vi "RunTest2.vi"(8 "error in (no error)":errorcluster, 11 "Prueba06 in":refnum<class "Prueba06.lvclass">) -> (0 "error out":errorcluster, 2 "resultado":string, 3 "Prueba06 out":refnum<class "Prueba06.lvclass">)   [LabVIEW 2019]
uses:
  Control/EstadosP06.ctl
  Prueba06.lvclass
  Control/MessageP06.ctl
  <vilib>/Utility/miscctls.llb/LVRowAndColumnTypeDef.ctl
  Prueba/Prueba.lvclass
  Prueba04/Control/Slide.ctl
  Prueba04/Prueba04.lvclass
  QMH/User Event - Stop/User Event - Stop.lvlib
  QMH/Message Queue/Message Queue.lvlib
  QMH/Message Queue/Enqueue Message (Single).vi
  ClusterGEN.ctl
  <vilib>/Utility/error.llb/Error Cluster From Error Code.vi
  <vilib>/ErrorRing/Error Ring.xnode
  <vilib>/Utility/error.llb/DialogType.ctl
  D:/REPO/GitHub/procal/Pruebas/Prueba/Prueba.lvclass
panel:
  out "tipoPrueba":string
  out "filaSelecc":i32
  out "TablaVoltajes":string[](array[string])
  out "cumple_no_cumple":bool
  out "n° filas":i32
  out "ptoCentral":dbl=2.0 format="%#.1f"
  out "Vref":dbl
  in  "Tab":enum32{"Page 1", "Page 2"}(tab)
  out "RangoRef":string
  out "frecuencia1":dbl=140.0
  in  "guardar_Vref":bool
  out "nivelRef":dbl=95.0 format="%.1f"
  in  "generar1":bool
  in  "AjusteAmp":T1=50.0 caption="Ajuste de amplitud [mV]" scale=0.0..20000.0
  out "voltaje1":dbl format="%.1f"
  out "frecuencia1":dbl format="%.1f"
  in  "seguir":bool
  out "Pict Ring 3":u16(ring)
  out "Pict Ring 2":u16(ring)
  in  "generar2":bool caption="PruebaSup"
  in  "PruebaInf":bool caption="PruebaSup"
  in  "PruebaSup":bool
  in  "Tabla":string[][](table)
  in  "salir":bool
  out "cumple":bool
  out "no_cumple":bool
  out "voltaje2":dbl format="%.1f"
  out "frecuencia2":dbl format="%.1f"
  in  "cb_rangoRef":string(combo)="1000"
  out "RangoRef2":string
  # "Elección Señal de Referencia\nsegún marca y modelo de sonómetro"
  # "Nivel Señal Referencia"
  # "Rango Referencia"
  # "Frecuencia"
  # "Monitoreo"
  # "Frecuencia"
  # "Hz"
  # "Voltaje"
  # "mV"
  # "6. Linealidad de nivel en el rango de referencia. IEC 61672-3: 2006 Cláusula 14"
  # "Tabla Resultados"
  # "Rango [dBA]"
  # "Referencia [dBA]"
  # "Cumple"
  # "No Cumple"
  # "6. Linealidad de nivel en el rango de referencia. IEC 61672-3: 2006 Cláusula 14"
  # "Monitoreo"
  # "Frecuencia"
  # "Hz"
  # "Voltaje"
  # "mV"
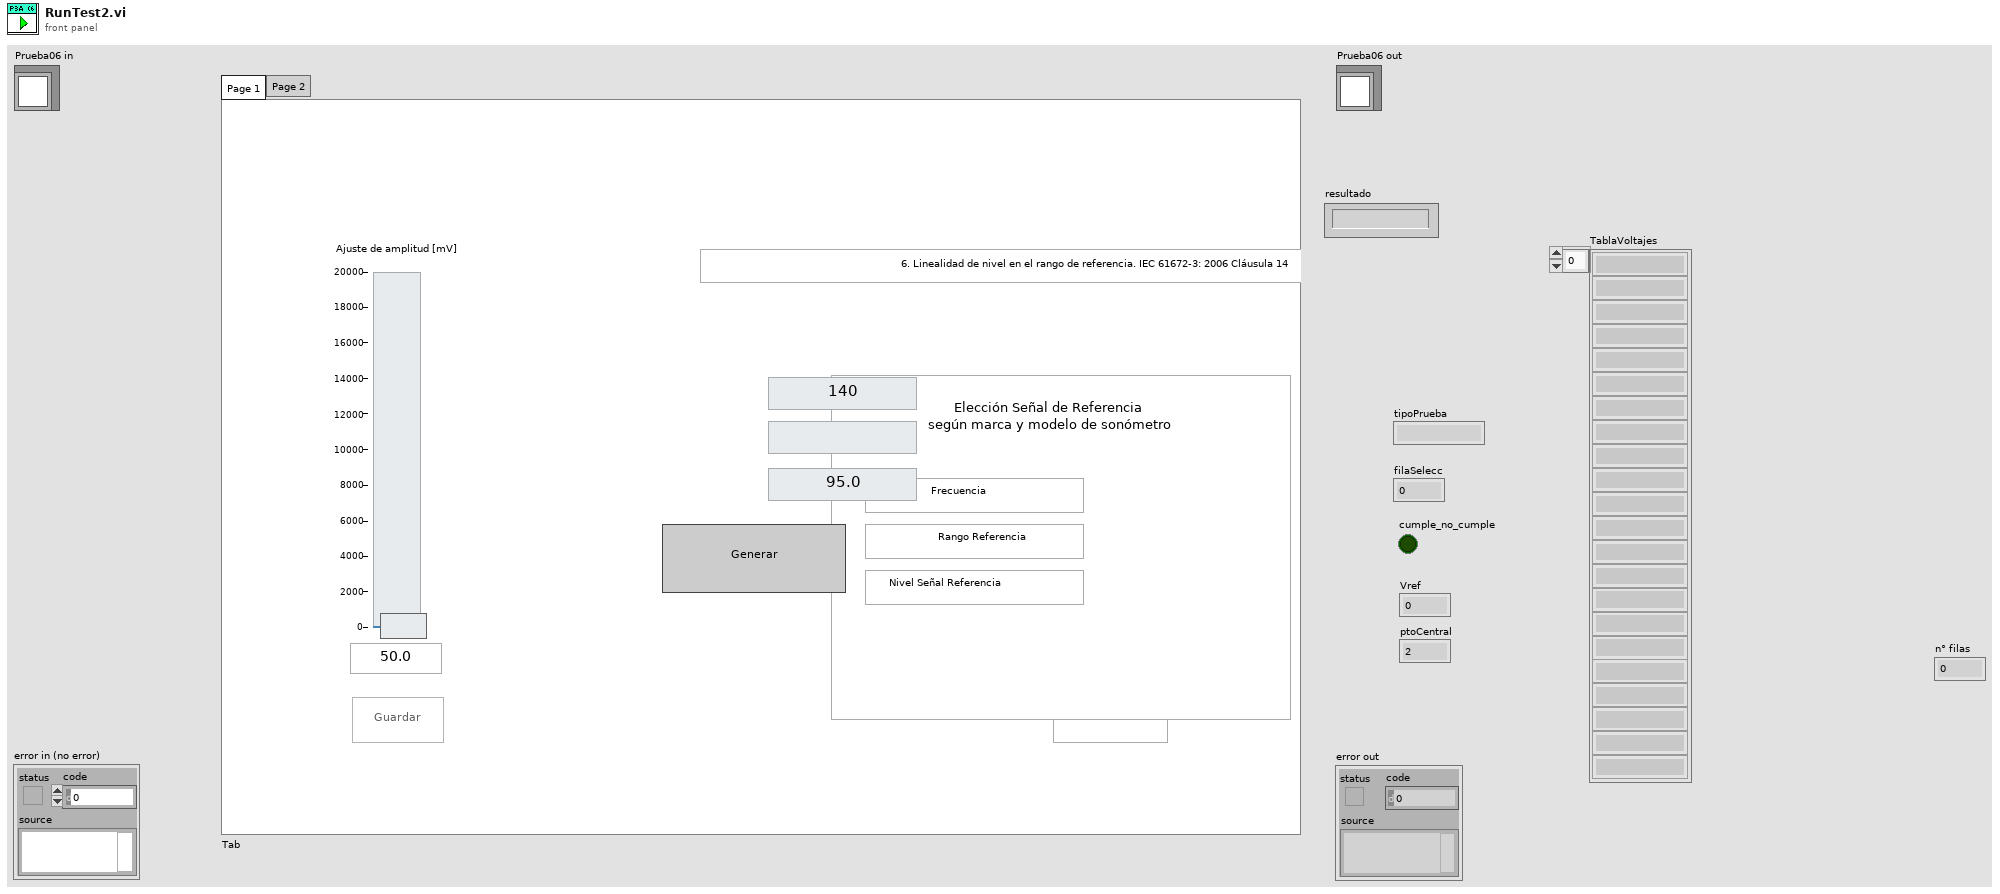
[diagram p1: front panel]
types:
  T1 = typedef "Prueba04.lvclass/Slide.ctl" = dbl
  T2 = typedef "LVRowAndColumnTypeDef.ctl" = cluster{"Row":i32, "Column":i32}
  T3 = typedef "Message Queue.lvlib/All Message Queues.ctl" = cluster{"MHL":refnum<queue>, "Inst_CNT90":refnum<queue>, "Inst_DS360":refnum<queue>, "Inst_Keithley2002":refnum<queue>, "Inst_DAQ":refnum<queue>, "BD":refnum<queue>, "Pistofono":refnum<queue>, "Nexus":refnum<queue>}
  T4 = enum8{"Enabled", "Disabled", "Disabled and Grayed Out"}
  T5 = typedef "Prueba06.lvclass/MessageP06.ctl" = cluster{"Estado":T6, "Data":variant}
  T6 = typedef "Prueba06.lvclass/EstadosP06.ctl" = enum16{"inicio", "LeerArchivoConfiguracion", "ConfirmarSalida", "DetieneInstrumentos", "InicializaInstrumento", "leerRango", "configuraRango", "calcularVref", "configuraTabla", "FrecAmp1", "FrecAmp2", "iniciarGEN", "monitoreo", "detenerGEN", "ajusteAmp", "guardaVerf", "creaVoltPrueba", "preguntaTipoPrueba", "guardarMediciones", "ingresaMediciones", "cumplimiento", "listo_evaluar", "evaluar", "final", "salir"}
  T7 = enum32{"Page 1", "Page 2", "Page 3", "Page 4", "Page 5", "Page 6", "Page 7"}
  T8 = typedef "Prueba06.lvclass/ClusterGEN.ctl" = cluster{"frec":dbl, "amp":dbl}
  T9 = cluster{"ControlName":string, "ControlReference":refnum<vi>}[]
  T10 = typedef "DialogType.ctl" = u16
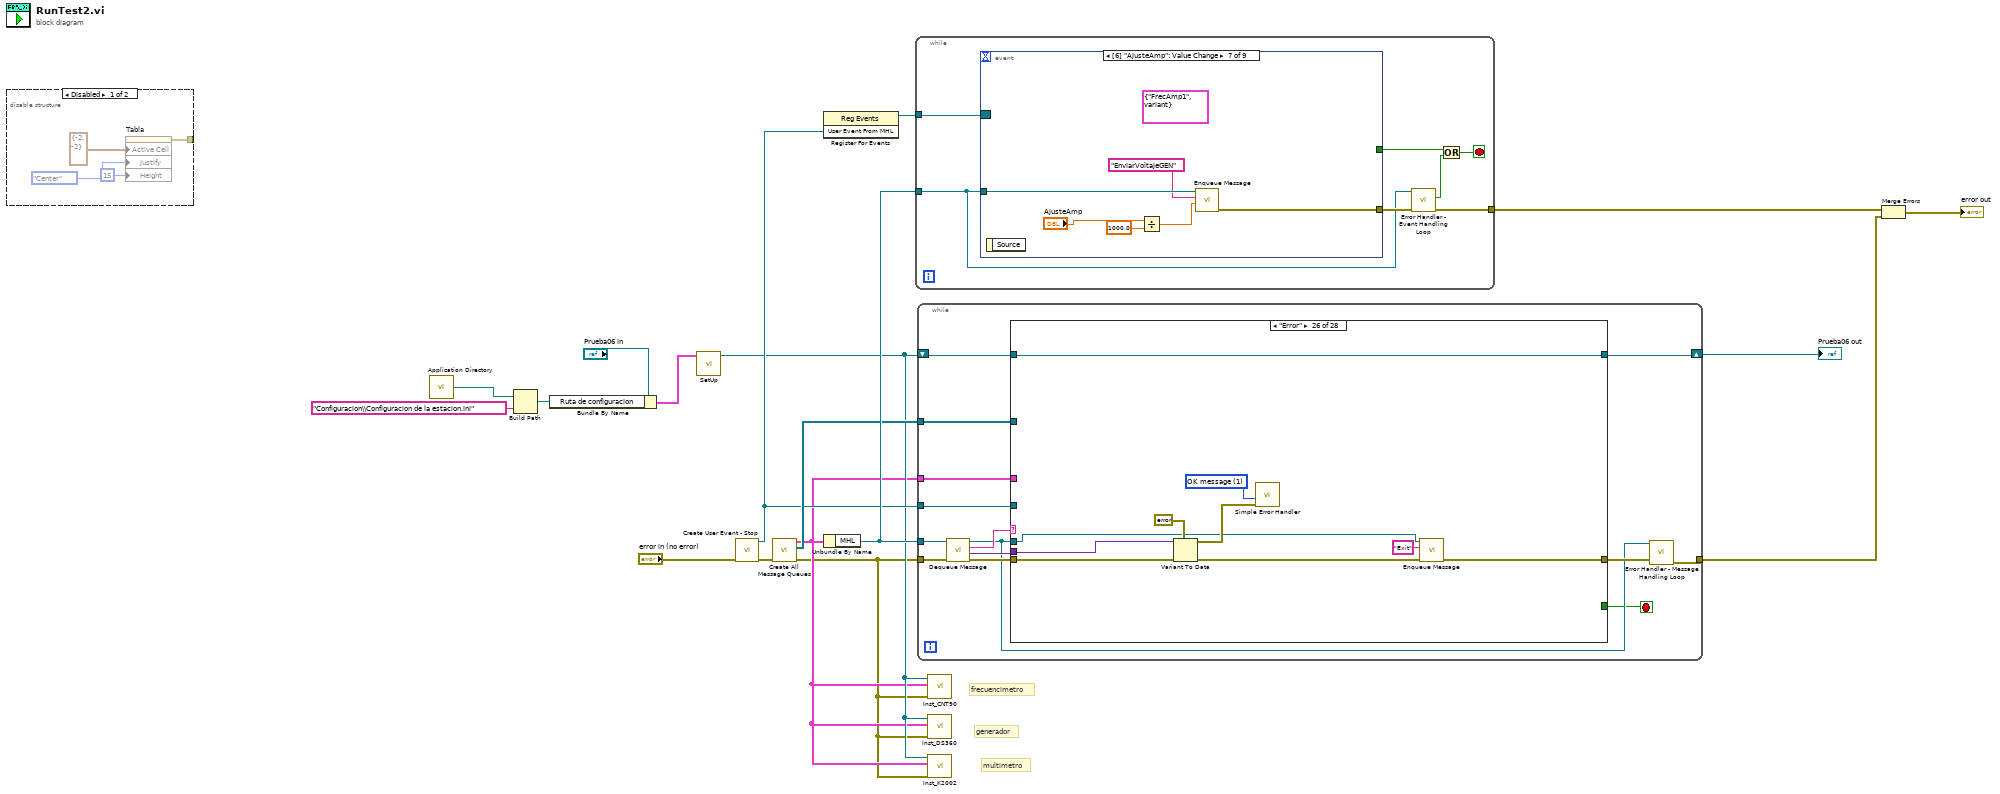
[diagram p0: block diagram]
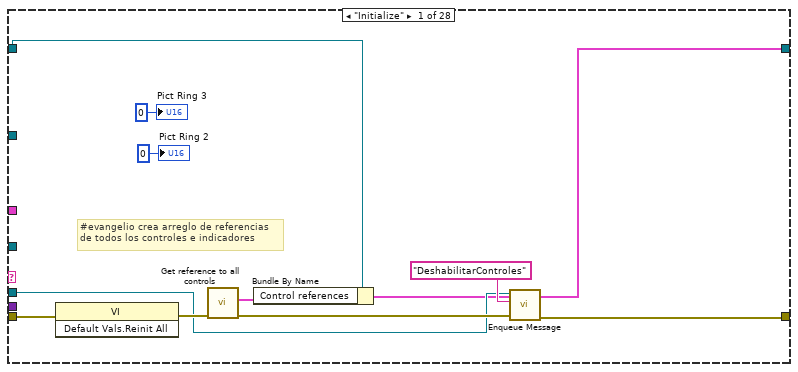
[diagram p3: hidden frame]
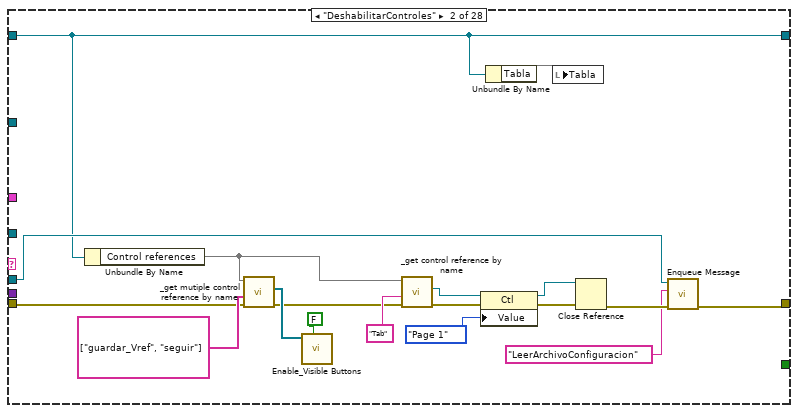
[diagram p4: hidden frame]
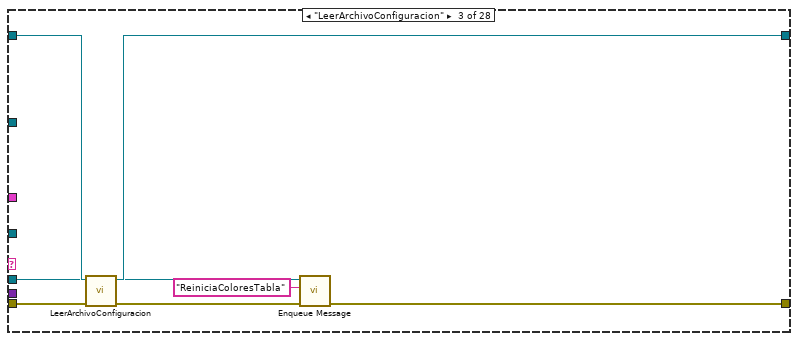
[diagram p5: hidden frame]
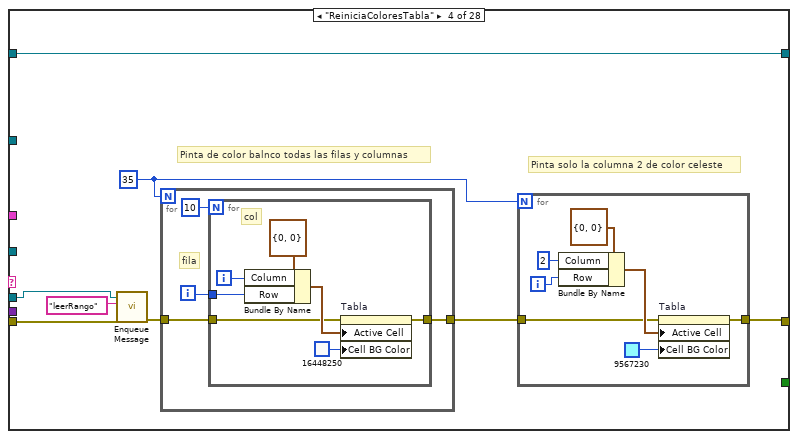
[diagram p6: hidden frame]
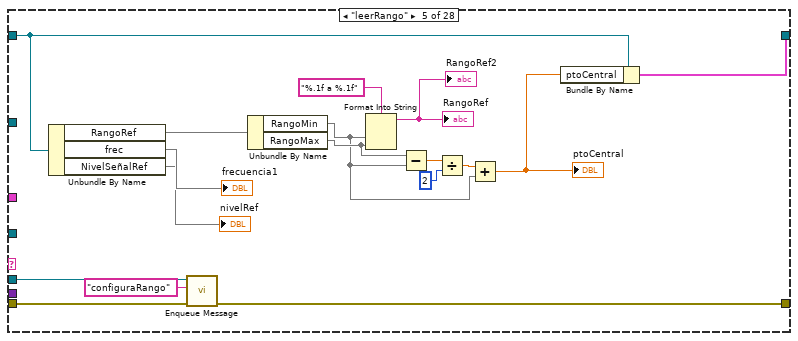
[diagram p7: hidden frame]
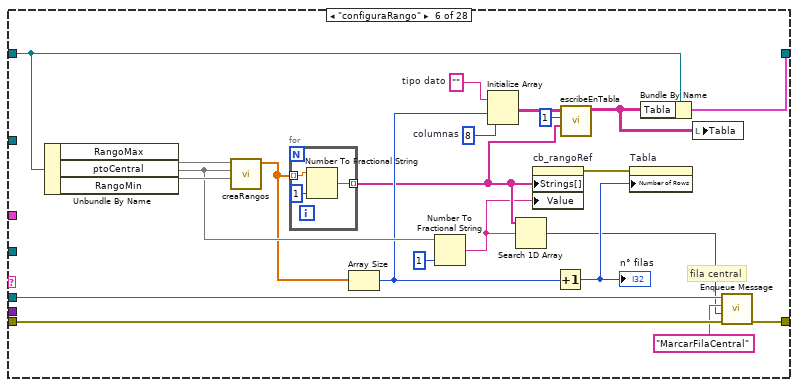
[diagram p8: hidden frame]
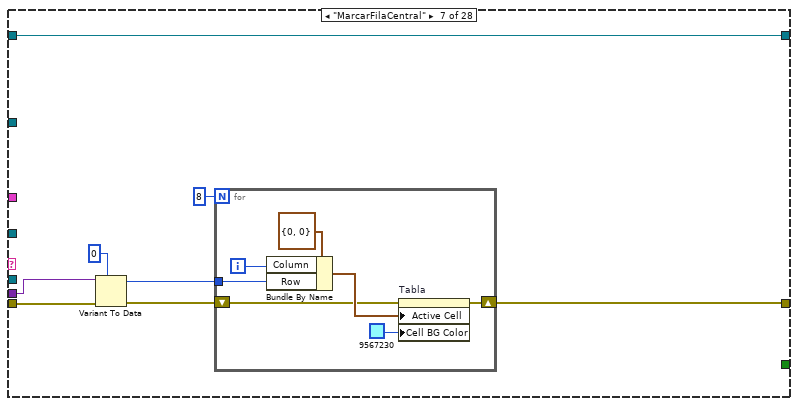
[diagram p9: hidden frame]
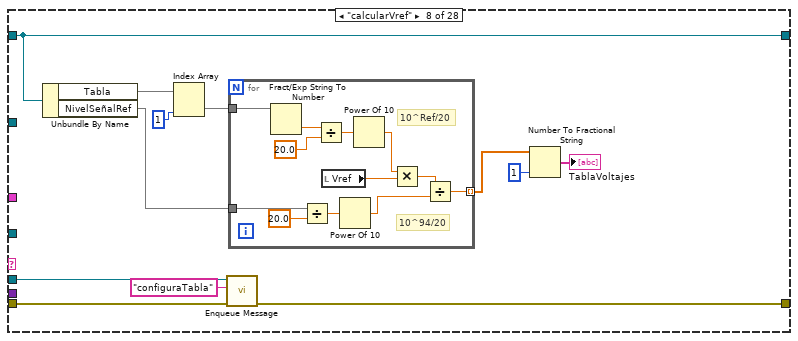
[diagram p10: hidden frame]
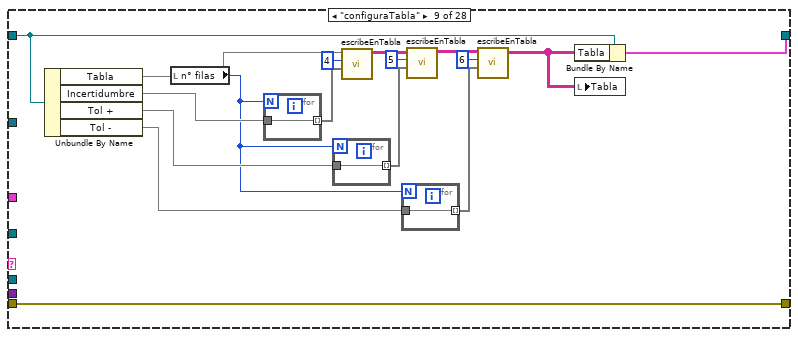
[diagram p11: hidden frame]
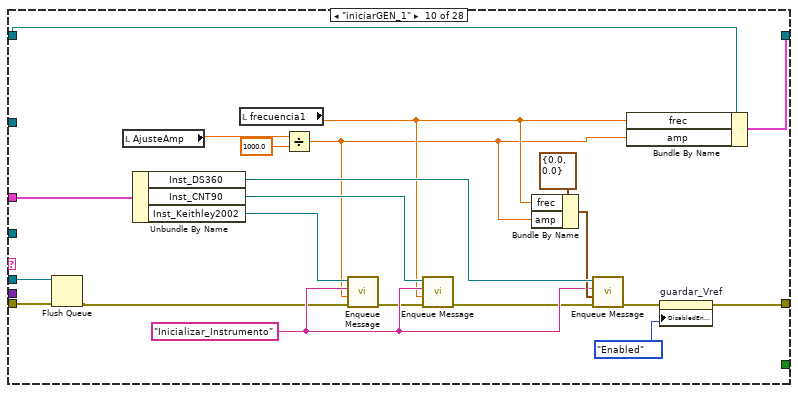
[diagram p12: hidden frame]
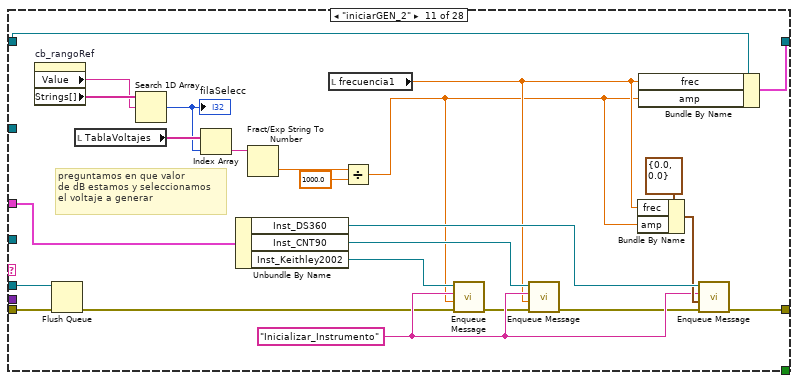
[diagram p13: hidden frame]
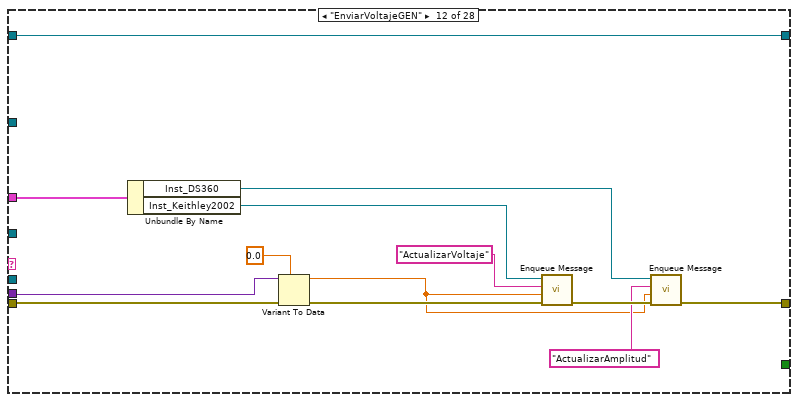
[diagram p14: hidden frame]
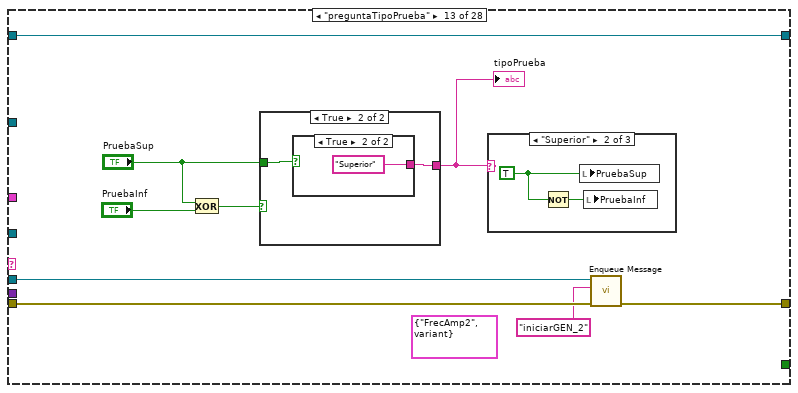
[diagram p15: hidden frame]
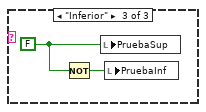
[diagram p17: hidden frame]
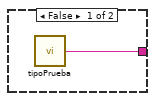
[diagram p18: hidden frame]
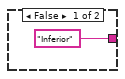
[diagram p19: hidden frame]
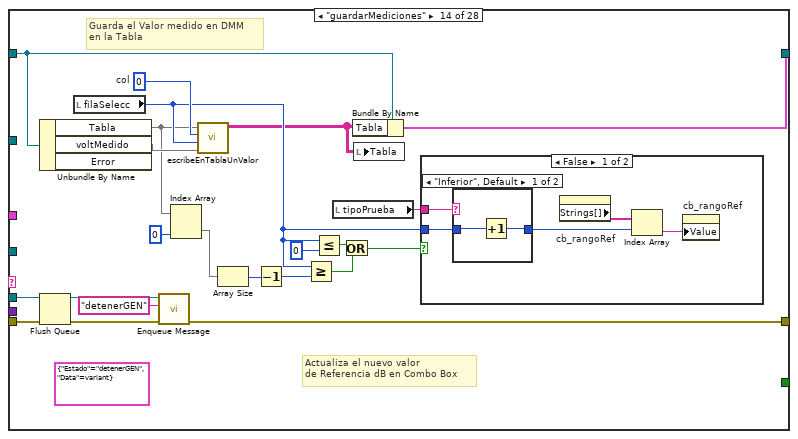
[diagram p20: hidden frame]
diagram:
  # "multimetro"
  # "generador"
  # "frecuencimetro"
  n1 = disable-structure shown="Disabled" {
    disable-tunnel: [w21 _] -> _
    frame Disabled {
      n2 = property on="Tabla" class="Tbl (strict)"("Active Cell"=T2 {"Row"=-2, "Column"=-2} ("Active Cell:Active Cell"), "Justify"=enum16{"Left", "Center", "Right"}."Center" ("Active Cell:Cell Justification"), "Height"=u32 15 ("Active Cell:Cell Font:Size")) -> (error out=w21:errorcluster)  [unwired: 2 in, 1 out]
    }
    frame Enabled {
    }
  }
  n3 = call <vilib>:"Application Directory.vi"() -> ("Application Directory"=w13:path)
  n4 = Build Path(base path=w13, name or relative path="Configuracion\\Configuracion de la estacion.ini") -> (appended path=w12:path)
  n5 = Bundle By Name(cluster="Prueba06 in", "Ruta de configuracion"=w12) -> (w10:cluster{})
  n6 = call-dynamic "SetUp.vi"("Prueba06 in"=w10) -> ("Prueba06 out"=w3:refnum<class "Prueba06.lvclass">)  [unwired: 9 in, 1 out]
  n7 = call "Create User Event - Stop.vi"("error in (no error)"="error in (no error)") -> ("error out"=w9:errorcluster, "User Event From MHL"=w5:refnum<user-event>)  [unwired: 9 in]
  n8 = call "Create All Message Queues.vi"("error in (no error)"=w9) -> ("error out"=w1:errorcluster, "PL Queues Array"=w6:refnum<queue>[], "All Message Queues out"=w2:T3)  [unwired: 8 in]
  n9 = register-events(w5) -> (reference out=w4:refnum<event-registration>)  [unwired: 2 in, 1 out]
  n10 = Unbundle By Name(w2) -> ("MHL"=w7:refnum<queue>)
  n11 = while {
    tunnel: w7 -> [w23]
    tunnel: [w27] -> w17
    tunnel: w4 -> [w25]
    stop <- w26 stop-if-true
    n12 = event shown="[6] \"AjusteAmp\": Value Change" {
      selector: w25 -> [_ _ _ _ _ _ _ _ _]
      dyn-events: _ -> [_ _ _ _ _ _ _ _ _]
      timeout: _ -> [_ _ _ _ _ _ _ _ _]
      tunnel: w23 -> [w32 _ w40 w47 w52 w58 w63 w69 w73]
      tunnel: [w31 _ _ w42 w53 w54 w64 w65 w72] -> w28
      tunnel: [_ w33 _ _ _ _ _ _ _] -> w24
      event "salir": Value Change {
        (unwired) T5 {"Estado"=enum."salir", "Data"=variant} ("element")
        n13 = event-data() -> ()  [unwired: 1 in, 1 out]
        n14 = call-poly "Enqueue Message.vi"("Message"="Exit", "Message Queue"=w32) -> ("error out"=w31:errorcluster)  [unwired: 8 in, 1 out]
      }
      event User Event {
        n15 = event-data() -> ("User Event"=w35:string, "Event Data"=w34:variant)  [unwired: 1 in]
        n16 = case shown="\"Exit EHL\"" w35 {
          tunnel: w34 -> [_ w37]
          tunnel: [_ w36] -> w33
          frame Default {
          }
          frame "Exit EHL" {
            # "#evangelio Termina\nla ejecucion del EHL"
            n17 = Variant To Data(type=TRUE, Variant=w37) -> (data=w36:bool)  [unwired: 1 in, 1 out]
          }
        }
      }
      event Panel Close? {
        w39 = TRUE
        n18 = event-data() -> ()  [unwired: 1 in, 1 out]
        n19 = call-poly "Enqueue Message.vi"("Priority Message? (F)"=w39, "Message"="Confirmar Salida", "Message Queue"=w40) -> ()  [unwired: 7 in, 2 out]
        n20 = event-data("Discard?"=w39) -> ()  [unwired: 1 in, 1 out]
      }
      event "generar1": Value Change {
        n21 = event-data() -> ("NewVal"=w46:bool)  [unwired: 1 in]
        n22 = Select(t="iniciarGEN_1", s=w46, f="detenerGEN") -> (s? t:f=w43:string)
        n23 = call-poly "Enqueue Message.vi"("Message"=w43, "Message Queue"=w47) -> ("error out"=w42:errorcluster)  [unwired: 8 in, 1 out]
      }
      event "generar2": Value Change {
        n24 = event-data() -> ("NewVal"=w51:bool)  [unwired: 1 in]
        n25 = Select(t="preguntaTipoPrueba", s=w51, f="guardarMediciones") -> (s? t:f=w48:string)
        n26 = call-poly "Enqueue Message.vi"("Message"=w48, "Message Queue"=w52) -> ("error out"=w53:errorcluster)  [unwired: 8 in, 1 out]
      }
      event "seguir": Value Change {
        (unwired) T5 {"Estado"=enum."calcularVref", "Data"=variant} ("element")
        n27 = event-data() -> ()  [unwired: 1 in, 1 out]
        n28 = call-poly "Enqueue Message.vi"("Message"="calcularVref", "Message Queue"=w58) -> ("error out"=w55:errorcluster)  [unwired: 8 in, 1 out]
        n29 = property on="Tab" class="TabCtl (strict)"(error in=w55, "Value"=enum32{"Page 1", "Page 2"}."Page 2" ("Tab")) -> (error out=w54:errorcluster)  [unwired: 1 in, 1 out]
      }
      event Value Change {
        (unwired) T5 {"Estado"=enum."FrecAmp1", "Data"=variant} ("element")
        n30 = event-data() -> ()  [unwired: 1 in, 1 out]
        n31 = Divide(x="AjusteAmp", y=T1 1000.0) -> (x/y=w59:T1)
        n32 = call-poly "Enqueue Message.vi"("Message Data"=w59, "Message"="EnviarVoltajeGEN", "Message Queue"=w63) -> ("error out"=w64:errorcluster)  [unwired: 7 in, 1 out]
      }
      event "guardar_Vref": Value Change {
        (unwired) T5 {"Estado"=enum."guardaVerf", "Data"=variant} ("element")
        n33 = event-data() -> ()  [unwired: 1 in, 1 out]
        n34 = call-poly "Enqueue Message.vi"("Message"="guardaVerf", "Message Queue"=w69) -> ("error out"=w66:errorcluster)  [unwired: 8 in, 1 out]
        n35 = property on="seguir" class="Bool"(error in=w66, "DisabledEnum"=T4."Enabled" ("Disabled")) -> (error out=w65:errorcluster)  [unwired: 1 in, 1 out]
      }
      event "Tabla": Value Change {
        n36 = event-data() -> ("NewVal"=w70:string[][])  [unwired: 1 in]
        n37 = call-poly "Enqueue Message.vi"("Message Data"=w70, "Message"="ingresaMediciones", "Message Queue"=w73) -> ("error out"=w72:errorcluster)  [unwired: 7 in, 1 out]
      }
    }
    n38 = call "Error Handler - Event Handling Loop.vi"("error in (no error)"=w28, "Message Queue"=w23) -> ("dup error in"=w27:errorcluster, "Error?"=w29:bool)  [unwired: 7 in, 1 out]
    n39 = Or(x=w24, y=w29) -> (x .or. y?=w26:bool)
  }
  n40 = while {
    tunnel: w7 -> [w85]
    tunnel: w1 -> [w84]
    tunnel: [w74] -> w16
    shift-right: [w86] -> w18
    shift-left: w3 -> [w87]
    tunnel: w2 -> [w79]
    tunnel: w6 -> [w78]
    tunnel: w5 -> [w80]
    stop <- w75 stop-if-true
    n41 = call "Dequeue Message.vi"("error in (no error)"=w84, "Message Queue"=w85) -> ("error out"=w83:errorcluster, "Message Data"=w81:variant, "Message"=w82:string, "dup Message Queue"=w76:refnum<queue>)  [unwired: 6 in]
    n42 = case shown="\"Error\"" w82 {
      selector: w82 -> [_ _ _ _ _ _ _ _ _ _ _ _ _ _ _ _ _ _ _ _ _ _ _ w472 _ _ _ w508]
      tunnel: [w91 w100 w121 w131 w165 w184 w199 w216 w240 w270 w294 w308 w317 w329 w360 w375 w383 w400 w418 w426 w431 w437 w465 w471 w489 w504 w506 w509] -> w86
      tunnel: w87 -> [w92 w100 w122 w131 w166 w186 w199 w216 w241 w271 w295 w308 w317 w347 w371 w379 w383 w400 w418 w429 w436 w437 w465 w471 w489 w504 w506 w509]
      tunnel: w81 -> [_ _ _ _ _ _ w197 _ _ _ _ w298 _ _ w364 _ _ _ _ w427 w433 _ _ _ _ w495 _ _]
      tunnel: w83 -> [w93 w102 w123 w129 w164 w178 w198 w214 w239 w269 w293 w299 w313 w348 w373 w381 w390 w403 w416 w428 w435 w439 w460 w473 w484 w498 w505 _]
      tunnel: [w90 w99 w118 w125 w155 w172 w194 w212 w239 w255 w275 w296 w312 w341 w370 w378 w389 w401 w416 w422 w434 w438 w460 w467 w482 w496 w505 w507] -> w77
      tunnel: [_ _ _ _ _ _ _ _ _ _ _ _ _ _ _ _ _ _ _ _ _ _ _ w468 _ _ _ _] -> w75
      tunnel: w76 -> [w94 w101 w119 w128 w154 w171 _ w213 _ w268 w292 _ w310 w344 w367 w377 w388 w402 _ _ _ w440 _ w466 w483 w497 _ _]
      tunnel: w80 -> [_ _ _ _ _ _ _ _ _ _ _ _ _ _ _ _ _ _ _ _ _ _ _ w469 _ _ _ _]
      tunnel: w79 -> [_ _ _ _ _ _ _ _ _ w251 w274 w297 _ _ _ _ _ _ _ _ _ w441 _ _ _ _ _ _]
      tunnel: w78 -> [_ _ _ _ _ _ _ _ _ _ _ _ _ _ _ _ _ _ _ _ _ _ _ w470 _ _ _ _]
      frame "Initialize" {
        # "#evangelio crea arreglo de referencias\nde todos los controles e indicadores"
        n43 = invoke class="VI" method="Default Vals.Reinit All"(error in=w93) -> (error out=w97:errorcluster)  [unwired: 2 in, 2 out]
        n44 = call "Get reference to all controls.vi"("error in (no error)"=w97) -> ("error out"=w95:errorcluster, "Control references"=w96:T9)  [unwired: 5 in]
        n45 = Bundle By Name(cluster=w92, "Control references"=w96) -> (w91:cluster{})
        n46 = call-poly "Enqueue Message.vi"("error in (no error)"=w95, "Message"="DeshabilitarControles", "Message Queue"=w94) -> ("error out"=w90:errorcluster)  [unwired: 7 in, 1 out]
        "Pict Ring 2" <- u16 0 ("Pict Ring 2")
        "Pict Ring 3" <- u16 0 ("Pict Ring 3")
      }
      frame "DeshabilitarControles" {
        n47 = Unbundle By Name(w100) -> ("Control references"=w111)
        n48 = call "_get mutiple control reference by name.vi"("error in (no error)"=w102, "Control names"=string[] ["guardar_Vref", "seguir"], "Control references"=w111) -> ("error out"=w108:errorcluster, "References"=w109:refnum<vi>[])  [unwired: 3 in]
        n49 = call "Enable_Visible Buttons.vi"("Enable? (T)"=FALSE, "Controls Ref Array"=w109) -> ()  [unwired: 10 in]
        n50 = call "_get control reference by name.vi"("error in (no error)"=w108, "Control name"="Tab" ("Message"), "Control references"=w111) -> ("error out"=w115:errorcluster, "Ctl Refnum"=w113:refnum<vi>)  [unwired: 3 in]
        n51 = property class="Ctl"(reference=w113, error in=w115, "Value"=T7."Page 1" ("Tab_Prueba04")) -> (reference out=w104:refnum<vi>, error out=w106:errorcluster)
        n52 = Unbundle By Name(w100) -> ("Tabla"=w116)
        n53 = local write "Tabla"(w116) -> ()
        n54 = Close Reference(reference=w104, error in (no error)=w106) -> (error out=w105:errorcluster)
        n55 = call-poly "Enqueue Message.vi"("error in (no error)"=w105, "Message"="LeerArchivoConfiguracion", "Message Queue"=w101) -> ("error out"=w99:errorcluster)  [unwired: 7 in, 1 out]
      }
      frame "LeerArchivoConfiguracion" {
        n56 = call "LeerArchivoConfiguracion.vi"("error in"=w123, "Prueba06 in"=w122) -> ("error out"=w120:errorcluster, "Prueba06 out"=w121:refnum<class "Prueba06.lvclass">)  [unwired: 8 in]
        n57 = call-poly "Enqueue Message.vi"("error in (no error)"=w120, "Message"="ReiniciaColoresTabla", "Message Queue"=w119) -> ("error out"=w118:errorcluster)  [unwired: 7 in, 1 out]
      }
      frame "ReiniciaColoresTabla" {
        w124 = 35
        # "Pinta solo la columna 2 de color celeste"
        # "Pinta de color balnco todas las filas y columnas"
        n58 = call-poly "Enqueue Message.vi"("error in (no error)"=w129, "Message"="leerRango", "Message Queue"=w128) -> ("error out"=w127:errorcluster)  [unwired: 7 in, 1 out]
        n59 = for {
          N: w124 -> [_]
          tunnel: w127 -> [w135]
          tunnel: [w134] -> w126
          i -> [w133]
          # "fila"
          n60 = for {
            N: 10 -> [_]
            tunnel: [w139] -> w134
            tunnel: w135 -> [w138]
            tunnel: w133 -> [w137]
            i -> [w136]
            # "col"
            n61 = Bundle By Name(cluster=T2 {"Row"=0, "Column"=0} ("Active Cell:Active Cell"), "Column"=w136, "Row"=w137) -> (w141:T2)
            n62 = property on="Tabla" class="Tbl (strict)"(error in=w138, "Active Cell"=w141, "Cell BG Color"=u32 16448250) -> (error out=w139:errorcluster)  [unwired: 1 in, 1 out]
          }
        }
        n63 = for {
          N: w124 -> [_]
          tunnel: [w145] -> w125
          tunnel: w126 -> [w143]
          i -> [w144]
          n64 = Bundle By Name(cluster=T2 {"Row"=0, "Column"=0} ("Active Cell:Active Cell"), "Column"=2, "Row"=w144) -> (w147:T2)
          n65 = property on="Tabla" class="Tbl (strict)"(error in=w143, "Active Cell"=w147, "Cell BG Color"=u32 9567230) -> (error out=w145:errorcluster)  [unwired: 1 in, 1 out]
        }
      }
      frame "leerRango" {
        n66 = Unbundle By Name(w166) -> ("RangoRef"=w163, "frec"=→"frecuencia1", "NivelSeñalRef"=→"nivelRef")
        n67 = call-poly "Enqueue Message.vi"("error in (no error)"=w164, "Message"="configuraRango", "Message Queue"=w154) -> ("error out"=w155:errorcluster)  [unwired: 7 in, 1 out]
        n68 = Unbundle By Name(w163) -> ("RangoMin"=w156, "RangoMax"=w161)
        n69 = Format Into String(format string="%.1f a %.1f", w156, w161) -> (resulting string=→"RangoRef" →"RangoRef2":string)  [unwired: 2 in, 1 out]
        n70 = Subtract(x=w161, y=w156) -> (x-y=w158:dbl)
        n71 = Divide(x=w158, y=u32 2) -> (x/y=w159:dbl)
        n72 = Add(x=w159, y=w156) -> (x+y=w160:dbl)
        "ptoCentral" <- w160
        n73 = Bundle By Name(cluster=w166, "ptoCentral"=w160) -> (w165:cluster{})
      }
      frame "configuraRango" {
        w177 = 8  # columnas
        w176 = ""  # tipo dato
        # "fila central"
        n74 = Unbundle By Name(w186) -> ("RangoMax"=w188, "ptoCentral"=w183, "RangoMin"=w187)
        n75 = call "creaRangos.vi"("RangoMin"=w187, "ptoCentral"=w183, "RangoMax"=w188) -> ("RangoCompleto"=w182:dbl[])  [unwired: 5 in, 3 out]
        n76 = for {
          tunnel: w182 -> [w191] mode=indexing
          tunnel: [w190] -> w169 mode=indexing
          n77 = Number To Fractional String(number=w191, precision (6)=i16 1) -> (F-format string=w190:string)  [unwired: 2 in]
        }
        n78 = Array Size(array=w182) -> (size(s)=w175:i32)
        n79 = Number To Fractional String(number=w183, precision (6)=i16 1) -> (F-format string=w168:string)  [unwired: 2 in]
        n80 = Initialize Array(w176, w175, w177) -> (w174:string[][])
        n81 = Search 1D Array(1D array=w169, element=w168) -> (index of element=w167:i32)  [unwired: 1 in]
        n82 = property on="cb_rangoRef" class="CmbBox"("Strings[]"=w169, "Value"=w168) -> (error out=w181:errorcluster)  [unwired: 2 in, 1 out]
        n83 = Increment(x=w175) -> (x+1=w180:i32)
        "n° filas" <- w180
        n84 = call "escribeEnTabla.vi"("parametros"=w169, "col"=1, "tabla in"=w174) -> ("tabla out"=w173:string[][])  [unwired: 8 in]
        n85 = property on="Tabla" class="Tbl (strict)"(error in=w181, "Number of Rows"=w180) -> ()  [unwired: 1 in, 2 out]
        n86 = Bundle By Name(cluster=w186, "Tabla"=w173) -> (w184:cluster{})
        n87 = local write "Tabla"(w173) -> ()
        n88 = call-poly "Enqueue Message.vi"("error in (no error)"=w178, "Message Data"=w167, "Message"="MarcarFilaCentral", "Message Queue"=w171) -> ("error out"=w172:errorcluster)  [unwired: 6 in, 1 out]
      }
      frame "MarcarFilaCentral" {
        n89 = Variant To Data(error in=w198, type=0, Variant=w197) -> (data=w193:i32, error out=w195:errorcluster)
        n90 = for {
          N: 8 -> [_]
          tunnel: w193 -> [w201]
          shift-right: [w202] -> w194
          shift-left: w195 -> [w203]
          i -> [w200]
          n91 = Bundle By Name(cluster=T2 {"Row"=0, "Column"=0} ("Active Cell:Active Cell"), "Column"=w200, "Row"=w201) -> (w205:T2)
          n92 = property on="Tabla" class="Tbl (strict)"(error in=w203, "Active Cell"=w205, "Cell BG Color"=u32 9567230) -> (error out=w202:errorcluster)  [unwired: 1 in, 1 out]
        }
      }
      frame "calcularVref" {
        n93 = Unbundle By Name(w216) -> ("Tabla"=w218, "NivelSeñalRef"=w211)
        n94 = Index Array(array=w218, index (col)=1 ("disabled index (col)")) -> (element=w209)  [unwired: 1 in]
        n95 = call-poly "Enqueue Message.vi"("error in (no error)"=w214, "Message"="configuraTabla", "Message Queue"=w213) -> ("error out"=w212:errorcluster)  [unwired: 7 in, 1 out]
        n96 = for {
          tunnel: w211 -> [w224]
          tunnel: [w221] -> w210 mode=indexing
          tunnel: w209 -> [w220]
          # "10^94/20"
          # "10^Ref/20"
          n97 = Fract/Exp String To Number(string=w220) -> (number=w230:dbl)  [unwired: 3 in, 1 out]
          n98 = Divide(x=w224, y=20.0) -> (x/y=w225:dbl)
          n99 = Divide(x=w230, y=20.0) -> (x/y=w228:dbl)
          n100 = local read "Vref"() -> (w219:dbl)
          n101 = Power Of 10(x=w225) -> (10^x=w222:dbl)
          n102 = Power Of 10(x=w228) -> (10^x=w227:dbl)
          n103 = Multiply(x=w227, y=w219) -> (x*y=w226:dbl)
          n104 = Divide(x=w226, y=w222) -> (x/y=w221:dbl)
        }
        n105 = Number To Fractional String(number=w210, precision (6)=i16 1) -> (F-format string=→"TablaVoltajes":string[])  [unwired: 2 in]
      }
      frame "configuraTabla" {
        n106 = Unbundle By Name(w241) -> ("Tabla"=w242, "Incertidumbre"=w238, "Tol +"=w236, "Tol -"=w235)
        n107 = local read "n° filas"() -> (w234:i32)
        n108 = for {
          N: w234 -> [_]
          tunnel: w238 -> [w250]
          tunnel: [w250] -> w237 mode=indexing
        }
        n109 = for {
          N: w234 -> [_]
          tunnel: w236 -> [w249]
          tunnel: [w249] -> w233 mode=indexing
        }
        n110 = call "escribeEnTabla.vi"("parametros"=w237, "col"=4, "tabla in"=w242) -> ("tabla out"=w247:string[][])  [unwired: 8 in]
        n111 = for {
          N: w234 -> [_]
          tunnel: w235 -> [w248]
          tunnel: [w248] -> w232 mode=indexing
        }
        n112 = call "escribeEnTabla.vi"("parametros"=w233, "col"=5, "tabla in"=w247) -> ("tabla out"=w246:string[][])  [unwired: 8 in]
        n113 = call "escribeEnTabla.vi"("parametros"=w232, "col"=6, "tabla in"=w246) -> ("tabla out"=w231:string[][])  [unwired: 8 in]
        n114 = Bundle By Name(cluster=w241, "Tabla"=w231) -> (w240:cluster{})
        n115 = local write "Tabla"(w231) -> ()
      }
      frame "iniciarGEN_1" {
        w261 = "Inicializar_Instrumento" ("Message")
        n116 = Flush Queue(queue=w268, error in (no error)=w269) -> (error out=w256:errorcluster)  [unwired: 2 out]
        n117 = local read "AjusteAmp"() -> (w267:T1)
        n118 = Unbundle By Name(w251) -> ("Inst_DS360"=w265:refnum<queue>, "Inst_CNT90"=w264:refnum<queue>, "Inst_Keithley2002"=w263:refnum<queue>)
        n119 = local read "frecuencia1"() -> (w253:dbl)
        n120 = Divide(x=w267, y=T1 1000.0) -> (x/y=w252:T1)
        n121 = call-poly "Enqueue Message.vi"("error in (no error)"=w256, "Message Data"=w252, "Message"=w261, "Message Queue"=w263) -> ("error out"=w260:errorcluster)  [unwired: 6 in, 1 out]
        n122 = call-poly "Enqueue Message.vi"("error in (no error)"=w260, "Message Data"=w253, "Message"=w261, "Message Queue"=w264) -> ("error out"=w259:errorcluster)  [unwired: 6 in, 1 out]
        n123 = Bundle By Name(cluster=T8 {"frec"=0.0, "amp"=0.0} ("clusterGEN"), "frec"=w253, "amp"=w252) -> (w262:T8)
        n124 = call-poly "Enqueue Message.vi"("error in (no error)"=w259, "Message Data"=w262, "Message"=w261, "Message Queue"=w265) -> ("error out"=w257:errorcluster)  [unwired: 6 in, 1 out]
        n125 = Bundle By Name(cluster=w271, "frec"=w253, "amp"=w252) -> (w270:cluster{})
        n126 = property on="guardar_Vref" class="Bool"(error in=w257, "DisabledEnum"=T4."Enabled" ("Disabled")) -> (error out=w255:errorcluster)  [unwired: 1 in, 1 out]
      }
      frame "iniciarGEN_2" {
        w280 = "Inicializar_Instrumento" ("Message")
        # "preguntamos en que valor \nde dB estamos y seleccionamos\nel voltaje a generar"
        n127 = property on="cb_rangoRef" class="CmbBox"() -> ("Value"=w290:string, "Strings[]"=w291:string[])  [unwired: 2 in, 2 out]
        n128 = Flush Queue(queue=w292, error in (no error)=w293) -> (error out=w276:errorcluster)  [unwired: 2 out]
        n129 = local read "TablaVoltajes"() -> (w289:string[])
        n130 = Search 1D Array(1D array=w291, element=w290) -> (index of element=w288:i32)  [unwired: 1 in]
        "filaSelecc" <- w288
        n131 = Index Array(array=w289, index=w288) -> (element=w287:string)
        n132 = Unbundle By Name(w274) -> ("Inst_DS360"=w284:refnum<queue>, "Inst_CNT90"=w283:refnum<queue>, "Inst_Keithley2002"=w282:refnum<queue>)
        n133 = Fract/Exp String To Number(string=w287) -> (number=w286:dbl)  [unwired: 3 in, 1 out]
        n134 = local read "frecuencia1"() -> (w273:dbl)
        n135 = Divide(x=w286, y=1000.0) -> (x/y=w272:dbl)
        n136 = call-poly "Enqueue Message.vi"("error in (no error)"=w276, "Message Data"=w272, "Message"=w280, "Message Queue"=w282) -> ("error out"=w279:errorcluster)  [unwired: 6 in, 1 out]
        n137 = call-poly "Enqueue Message.vi"("error in (no error)"=w279, "Message Data"=w273, "Message"=w280, "Message Queue"=w283) -> ("error out"=w278:errorcluster)  [unwired: 6 in, 1 out]
        n138 = Bundle By Name(cluster=T8 {"frec"=0.0, "amp"=0.0} ("clusterGEN"), "frec"=w273, "amp"=w272) -> (w281:T8)
        n139 = Bundle By Name(cluster=w295, "frec"=w273, "amp"=w272) -> (w294:cluster{})
        n140 = call-poly "Enqueue Message.vi"("error in (no error)"=w278, "Message Data"=w281, "Message"=w280, "Message Queue"=w284) -> ("error out"=w275:errorcluster)  [unwired: 6 in, 1 out]
      }
      frame "EnviarVoltajeGEN" {
        n141 = Unbundle By Name(w297) -> ("Inst_DS360"=w302:refnum<queue>, "Inst_Keithley2002"=w307:refnum<queue>)
        n142 = Variant To Data(error in=w299, type=0.0, Variant=w298) -> (data=w300:dbl, error out=w305:errorcluster)
        n143 = call-poly "Enqueue Message.vi"("error in (no error)"=w305, "Message Data"=w300, "Message"="ActualizarVoltaje", "Message Queue"=w307) -> ("error out"=w303:errorcluster)  [unwired: 6 in, 1 out]
        n144 = call-poly "Enqueue Message.vi"("error in (no error)"=w303, "Message Data"=w300, "Message"="ActualizarAmplitud", "Message Queue"=w302) -> ("error out"=w296:errorcluster)  [unwired: 6 in, 1 out]
      }
      frame "preguntaTipoPrueba" {
        (unwired) T5 {"Estado"=enum."FrecAmp2", "Data"=variant} ("element")
        n145 = Exclusive Or(1:"PruebaInf", 2:"PruebaSup") -> (0:w316:bool)
        n146 = case shown="True" w316 {
          tunnel: "PruebaSup" -> [_ w324]
          tunnel: [w322 w323] -> w311
          frame False {
            n147 = call "tipoPrueba.vi"() -> ("tipoPrueba"=w322:string)  [unwired: 1 in]
          }
          frame True {
            n148 = case shown="True" w324 {
              tunnel: ["Inferior" "Superior"] -> w323
              frame False {
              }
              frame True {
              }
            }
          }
        }
        "tipoPrueba" <- w311
        n149 = case shown="\"Superior\"" w311 {
          frame Default {
          }
          frame "Superior" {
            w319 = TRUE ("PruebaSup")
            n150 = Not(x=w319) -> (.not. x?=w318:bool)
            n151 = local write "PruebaSup"(w319) -> ()
            n152 = local write "PruebaInf"(w318) -> ()
          }
          frame "Inferior" {
            w321 = FALSE ("PruebaSup")
            n153 = Not(x=w321) -> (.not. x?=w320:bool)
            n154 = local write "PruebaSup"(w321) -> ()
            n155 = local write "PruebaInf"(w320) -> ()
          }
        }
        n156 = call-poly "Enqueue Message.vi"("error in (no error)"=w313, "Message"="iniciarGEN_2", "Message Queue"=w310) -> ("error out"=w312:errorcluster)  [unwired: 7 in, 1 out]
      }
      frame "guardarMediciones" {
        (unwired) T5 {"Estado"=enum."detenerGEN", "Data"=variant} ("element")
        w346 = 0  # col
        # "Actualiza el nuevo valor\nde Referencia dB en Combo Box"
        # "Guarda el Valor medido en DMM\nen la Tabla"
        n157 = Unbundle By Name(w347) -> ("Tabla"=w334, "voltMedido"=w345)  [unwired: 1 out]
        n158 = Flush Queue(queue=w344, error in (no error)=w348) -> (queue out=w343:refnum<queue>, error out=w342:errorcluster)  [unwired: 1 out]
        n159 = local read "filaSelecc"() -> (w338:i32)
        n160 = call-poly "Enqueue Message.vi"("error in (no error)"=w342, "Message"="detenerGEN", "Message Queue"=w343) -> ("error out"=w341:errorcluster)  [unwired: 7 in, 1 out]
        n161 = Index Array(array=w334, index (col)=0 ("disabled index (col)")) -> (element=w332)  [unwired: 1 in]
        n162 = call "escribeEnTablaUnValor.vi"("element"=w345, "fila"=w338, "col"=w346, "tabla in"=w334) -> ("tabla out"=w328:string[][])  [unwired: 7 in]
        n163 = Array Size(array=w332) -> (size(s)=w336:i32)
        n164 = Decrement(x=w336) -> (x-1=w335:i32)
        n165 = Greater Or Equal?(x=w338, y=w335) -> (x >= y?=w337:bool)
        n166 = Less Or Equal?(x=w338, y=0) -> (x <= y?=w331:bool)
        n167 = local read "tipoPrueba"() -> (w340:string)
        n168 = Or(x=w331, y=w337) -> (x .or. y?=w330:bool)
        n169 = Bundle By Name(cluster=w347, "Tabla"=w328) -> (w329:cluster{})
        n170 = local write "Tabla"(w328) -> ()
        n171 = case shown="False" w330 {
          tunnel: w340 -> [w350 _]
          tunnel: w338 -> [w349 _]
          frame False {
            n172 = case shown="\"Inferior\", Default" w350 {
              tunnel: w349 -> [w355 w357]
              tunnel: [w354 w356] -> w353
              frame "Inferior", Default {
                n173 = Increment(x=w355) -> (x+1=w354:i32)
              }
              frame "Superior" {
                n174 = Decrement(x=w357) -> (x-1=w356:i32)
              }
            }
            n175 = property on="cb_rangoRef" class="CmbBox"() -> ("Strings[]"=w352:string[])  [unwired: 2 in, 2 out]
            n176 = Index Array(array=w352, index=w353) -> (element=w351:string)
            n177 = property on="cb_rangoRef" class="CmbBox"("Value"=w351) -> ()  [unwired: 2 in, 2 out]
          }
          frame True {
            n178 = One Button Dialog(message="Llegamos al final de la Tabla") -> ()  [unwired: 1 in, 1 out]
          }
        }
      }
      frame "ingresaMediciones" {
        (unwired) T5 {"Estado"=enum."cumplimiento", "Data"=variant} ("element")
        n179 = Flush Queue(queue=w367, error in (no error)=w373) -> (queue out=w366:refnum<queue>, error out=w368:errorcluster)  [unwired: 1 out]
        n180 = Variant To Data(error in=w368, type=string[][] [] ("NewVal"), Variant=w364) -> (data=w362:string[][], error out=w365:errorcluster)
        n181 = control-ref of="Tabla"() -> (w369:refnum<vi>)
        n182 = call "ingresaMediciones.vi"("error in (no error)"=w365, "Tbl Refnum"=w369, "New Value"=w362, "Prueba06 in"=w371) -> ("error out"=w372:errorcluster, "Prueba06 out"=w360:refnum<class "Prueba06.lvclass">)  [unwired: 6 in]
        n183 = Unbundle By Name(w360) -> ("Tabla"=w361)
        n184 = local write "Tabla"(w361) -> ()
        n185 = call-poly "Enqueue Message.vi"("error in (no error)"=w372, "Message"="cumplimiento", "Message Queue"=w366) -> ("error out"=w370:errorcluster)  [unwired: 7 in, 1 out]
      }
      frame "cumplimiento" {
        (unwired) T5 {"Estado"=enum."listo_evaluar", "Data"=variant} ("element")
        n186 = call "cumplimiento.vi"("error in (no error)"=w381, "Prueba06 in"=w379) -> ("error out"=w380:errorcluster, "Prueba06 out"=w375:refnum<class "Prueba06.lvclass">)  [unwired: 8 in]
        n187 = Unbundle By Name(w375) -> ("Tabla"=w376)
        n188 = local write "Tabla"(w376) -> ()
        n189 = call-poly "Enqueue Message.vi"("error in (no error)"=w380, "Message"="listo_evaluar", "Message Queue"=w377) -> ("error out"=w378:errorcluster)  [unwired: 7 in, 1 out]
      }
      frame "listo_evaluar" {
        n190 = Unbundle By Name(w383) -> ("Tabla"=w384)
        n191 = Index Array(array=w384, index (col)=7 ("disabled index (col)")) -> (element=w386)  [unwired: 1 in]
        n192 = for {
          tunnel: [w398] -> w385 mode=indexing
          tunnel: w386 -> [w396]
          n193 = Not Equal?(x=w396, y="") -> (x != y?=w398:bool)
        }
        n194 = And Array Elements(Boolean array=w385) -> (logical AND=w382:bool)
        n195 = case shown="True" w382 {
          tunnel: w390 -> [w391 w395]
          tunnel: [w391 w394] -> w389
          tunnel: w388 -> [_ w393]
          frame False {
          }
          frame True {
            n196 = call-poly "Enqueue Message.vi"("error in (no error)"=w395, "Message"="evaluar", "Message Queue"=w393) -> ("error out"=w394:errorcluster)  [unwired: 7 in, 1 out]
          }
        }
      }
      frame "evaluar" {
        (unwired) T5 {"Estado"=enum."final", "Data"=variant} ("element")
        # "si todos cumplen\nentonces el ensayo\ncumple"
        n197 = Unbundle By Name(w400) -> ("Tabla"=w404)
        n198 = Index Array(array=w404, index (col)=7 ("disabled index (col)")) -> (element=w406)  [unwired: 1 in]
        n199 = for {
          tunnel: [w411] -> w407 mode=indexing
          tunnel: w406 -> [w409]
          n200 = Equal?(x=w409, y="Cumple") -> (x = y?=w411:bool)
        }
        n201 = And Array Elements(Boolean array=w407) -> (logical AND=→"cumple_no_cumple":bool)
        n202 = call-poly "Enqueue Message.vi"("error in (no error)"=w403, "Message"="final", "Message Queue"=w402) -> ("error out"=w401:errorcluster)  [unwired: 7 in, 1 out]
      }
      frame "final" {
        n203 = local read "cumple_no_cumple"() -> (w412:bool)
        "cumple" <- w412
        n204 = Not(x=w412) -> (.not. x?=→"no_cumple":bool)
        n205 = Select(t="Cumple", s=w412, f="No Cumple") -> (s? t:f=→"resultado":string)
      }
      frame "DatoRecibidoK2002" {
        n206 = Variant To Data(error in=w428, type=0.0 ("y"), Variant=w427) -> (data=w420:dbl, error out=w422:errorcluster)
        n207 = Multiply(x=w420, y=1000.0) -> (x*y=w419:dbl)
        "voltaje1" <- w419
        n208 = Multiply(x=w420, y=1000.0) -> (x*y=→"voltaje2":dbl)
        n209 = Bundle By Name(cluster=w429, "voltMedido"=w419) -> (w426:cluster{})
      }
      frame "DatoRecibidoCNT90" {
        n210 = Variant To Data(error in=w435, type=0.0, Variant=w433) -> (data=w430:dbl, error out=w434:errorcluster)
        "frecuencia2" <- w430
        "frecuencia1" <- w430
        n211 = Bundle By Name(cluster=w436, "frecMedida"=w430) -> (w431:cluster{})
      }
      frame "detenerGEN" {
        w452 = TRUE ("Priority Message? (F)")
        w453 = "Detener_Instrumento"
        w458 = 0.0 ("voltaje1")
        n212 = Unbundle By Name(w441) -> ("Inst_DS360"=w454:refnum<queue>, "Inst_CNT90"=w455:refnum<queue>, "Inst_Keithley2002"=w456:refnum<queue>)
        n213 = Flush Queue(queue=w440, error in (no error)=w439) -> (error out=w457:errorcluster)  [unwired: 2 out]
        n214 = local write "voltaje1"(w458) -> ()
        n215 = local write "voltaje2"(w458) -> ()
        n216 = local write "frecuencia1"(w458) -> ()
        n217 = local write "frecuencia2"(w458) -> ()
        n218 = call-poly "Enqueue Message.vi"("Priority Message? (F)"=w452, "Message"=w453, "Message Queue"=w456) -> ()  [unwired: 7 in, 2 out]
        n219 = call-poly "Enqueue Message.vi"("Priority Message? (F)"=w452, "Message"=w453, "Message Queue"=w455) -> ()  [unwired: 7 in, 2 out]
        n220 = call-poly "Enqueue Message.vi"("Priority Message? (F)"=w452, "error in (no error)"=w457, "Message"=w453, "Message Queue"=w454) -> ("error out"=w450:errorcluster)  [unwired: 6 in, 1 out]
        n221 = Unbundle By Name(w437) -> ("Control references"=w445)
        n222 = Build Array("seguir" ("String")) -> (w442:string[])
        n223 = call-poly "get control reference by name.vi"("error in (no error)"=w450, "Control name"="guardar_Vref" ("String"), "Control references"=w445) -> ("error out"=w438:errorcluster, "Ctl Refnum"=w448:refnum<vi>)  [unwired: 3 in]
        n224 = Build Array(w448) -> (w447:refnum<vi>[])
        n225 = call-poly "get control reference by name.vi"("Control names"=w442, "Control references"=w445) -> ("References"=w444:refnum<vi>[])  [unwired: 4 in, 1 out]
        n226 = call "Enable_Visible Buttons.vi"("Enable? (T)"=FALSE, "Controls Ref Array"=w447) -> ()  [unwired: 10 in]
        n227 = call "Enable_Visible Buttons.vi"("Enable? (T)"=TRUE, "Controls Ref Array"=w444) -> ()  [unwired: 10 in]
      }
      frame "guardaVerf" {
        n228 = local read "AjusteAmp"() -> (w459:T1)
        "Vref" <- w459
        n229 = Number To Fractional String(number=w459, precision (6)=i16 3) -> (F-format string=w461:string)  [unwired: 2 in]
        n230 = Format Into String(format string="Se guardó Vref = %s volts", w461) -> (resulting string=w464:string)  [unwired: 2 in, 1 out]
        n231 = One Button Dialog(message=w464) -> ()  [unwired: 1 in, 1 out]
      }
      frame "Exit" {
        w468 = TRUE
        # "#evangelio Manda a cerrar el EHL"
        # "#evangelio Manda a cerrar todos los Loops"
        n232 = Release Queue(queue=w466, error in (no error)=w473) -> (error out=w477:errorcluster)  [unwired: 1 in, 2 out]
        n233 = Unbundle By Name(w471) -> ("Control references"=w478)
        n234 = for {
          tunnel: w470 -> [w481] mode=indexing
          tunnel: w472 -> [w480]
          tunnel: TRUE -> [w479]
          n235 = call-poly "Enqueue Message.vi"("Priority Message? (F)"=w479, "Message"=w480, "Message Queue"=w481) -> ()  [unwired: 7 in, 2 out]
        }
        n236 = call "Close All Ref.vi"("error in (no error)"=w477, "Control references"=w478) -> ("error out"=w475:errorcluster)  [unwired: 9 in]
        n237 = call "Fire User Event - Stop.vi"("error in (no error)"=w475, "Event Data"=w468, "User Event"="Exit EHL", "User Event in"=w469) -> ("error out"=w467:errorcluster)  [unwired: 7 in]
      }
      frame "Confirmar Salida" {
        n238 = Two Button Dialog(message="¿Quieres cerrar la aplicación?", 1:"No" ("T button name (\"OK\")"), 2:"Si" ("T button name (\"OK\")")) -> (T button?=w485:bool)
        n239 = case shown="True" w485 {
          tunnel: w484 -> [w490 w494]
          tunnel: [w490 w493] -> w482
          tunnel: w483 -> [_ w491]
          frame False {
          }
          frame True {
            n240 = call-poly "Enqueue Message.vi"("error in (no error)"=w494, "Message"="Exit", "Message Queue"=w491) -> ("error out"=w493:errorcluster)  [unwired: 7 in, 1 out]
          }
        }
      }
      frame "Error" {
        w502 = T10 1 items=["no dialog", "OK message", "continue or stop message", "OK message + warnings", "continue/stop + warnings"] ("type of dialog (OK msg:1)")
        n241 = Variant To Data(error in=w498, type=errorcluster {"status"=FALSE, "code"=0, "source"=""} ("error out"), Variant=w495) -> (data=w500:errorcluster, error out=w499:errorcluster)
        n242 = call <vilib>:"Simple Error Handler.vi"("type of dialog (OK msg:1)"=w502, "error in (no error)"=w500) -> ()  [unwired: 3 in, 5 out]
        n243 = call-poly "Enqueue Message.vi"("error in (no error)"=w499, "Message"="Exit", "Message Queue"=w497) -> ("error out"=w496:errorcluster)  [unwired: 7 in, 1 out]
      }
      frame "----------------------Controles----------------------" {
      }
      frame Default {
        n244 = xnode "Error Ring"("parameter 0"=w508) -> ("error out"=w507:errorcluster)
      }
    }
    n245 = call "Error Handler - Message Handling Loop.vi"("error in (no error)"=w77, "Message Queue"=w76) -> ("dup error in"=w74:errorcluster)  [unwired: 8 in, 1 out]
  }
  "Prueba06 out" <- w18
  n246 = call "Inst_CNT90.vi"("error in"=w1, "All Message Queues in"=w2, "Prueba31 in"=w3) -> ()  [unwired: 8 in, 1 out]
  n247 = call "Inst_DS360.vi"("error in"=w1, "All Message Queues in"=w2, "Prueba06 in"=w3) -> ()  [unwired: 8 in, 1 out]
  n248 = call "Inst_K2002.vi"("error in"=w1, "All Message Queues in"=w2, "Prueba31 in"=w3) -> ()  [unwired: 8 in, 1 out]
  n249 = Merge Errors(w17, w16) -> (→"error out":errorcluster)
